vi "mono_radar.vi"(7 "Sensor Connections":T1(array[cluster])) -> (0 "error out":errorcluster, 1 "radar_data_cube":csg[][][](array[numeric]), 2 "Sensor Connections Out":T1(array[cluster]), 3 "connection ID out":refnum<k5>)   [LabVIEW 2018]
panel:
  in  "n_sweeps":i32=64
  in  "n_elements":i32=8
  in  "samples_per_sweep":i32=825
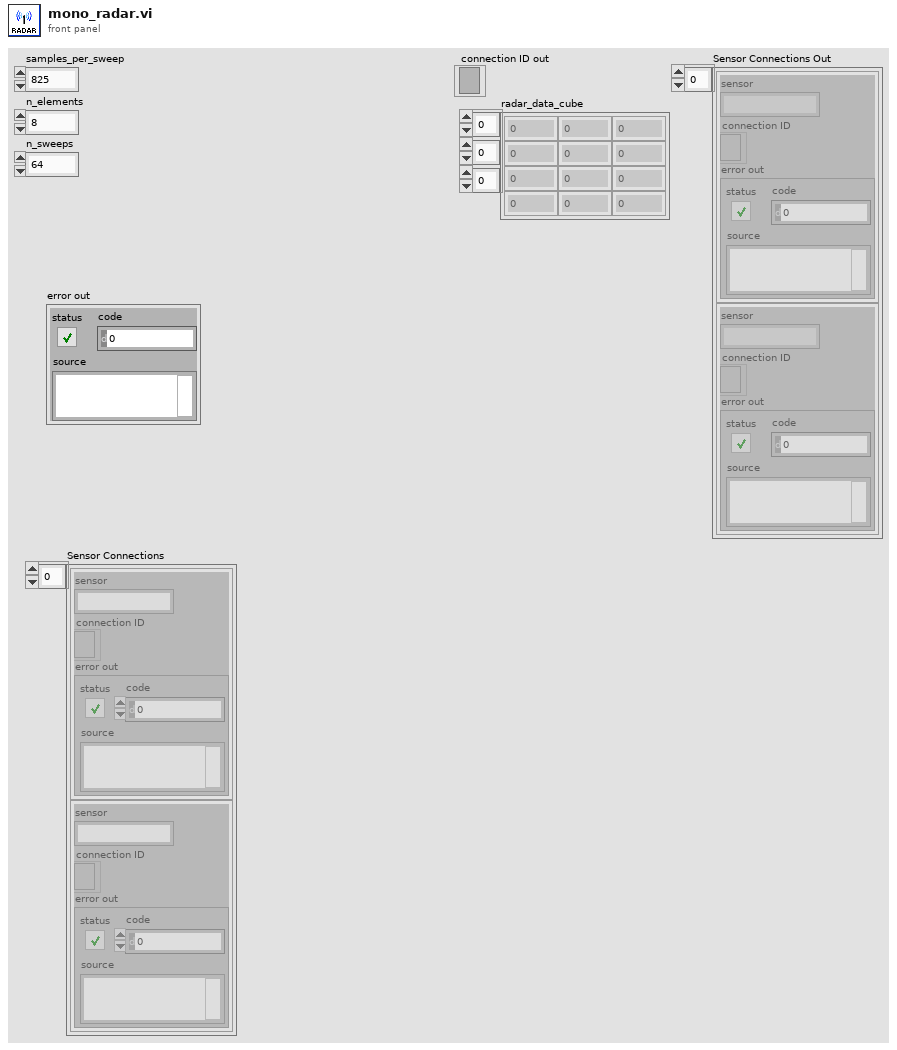
[diagram p1: front panel]
types:
  T1 = cluster{"sensor":string, "connection ID":refnum<k5>, "error out":errorcluster}[]
  T2 = cluster{"sensor":string, "connection ID":refnum<k5>, "error out":errorcluster}
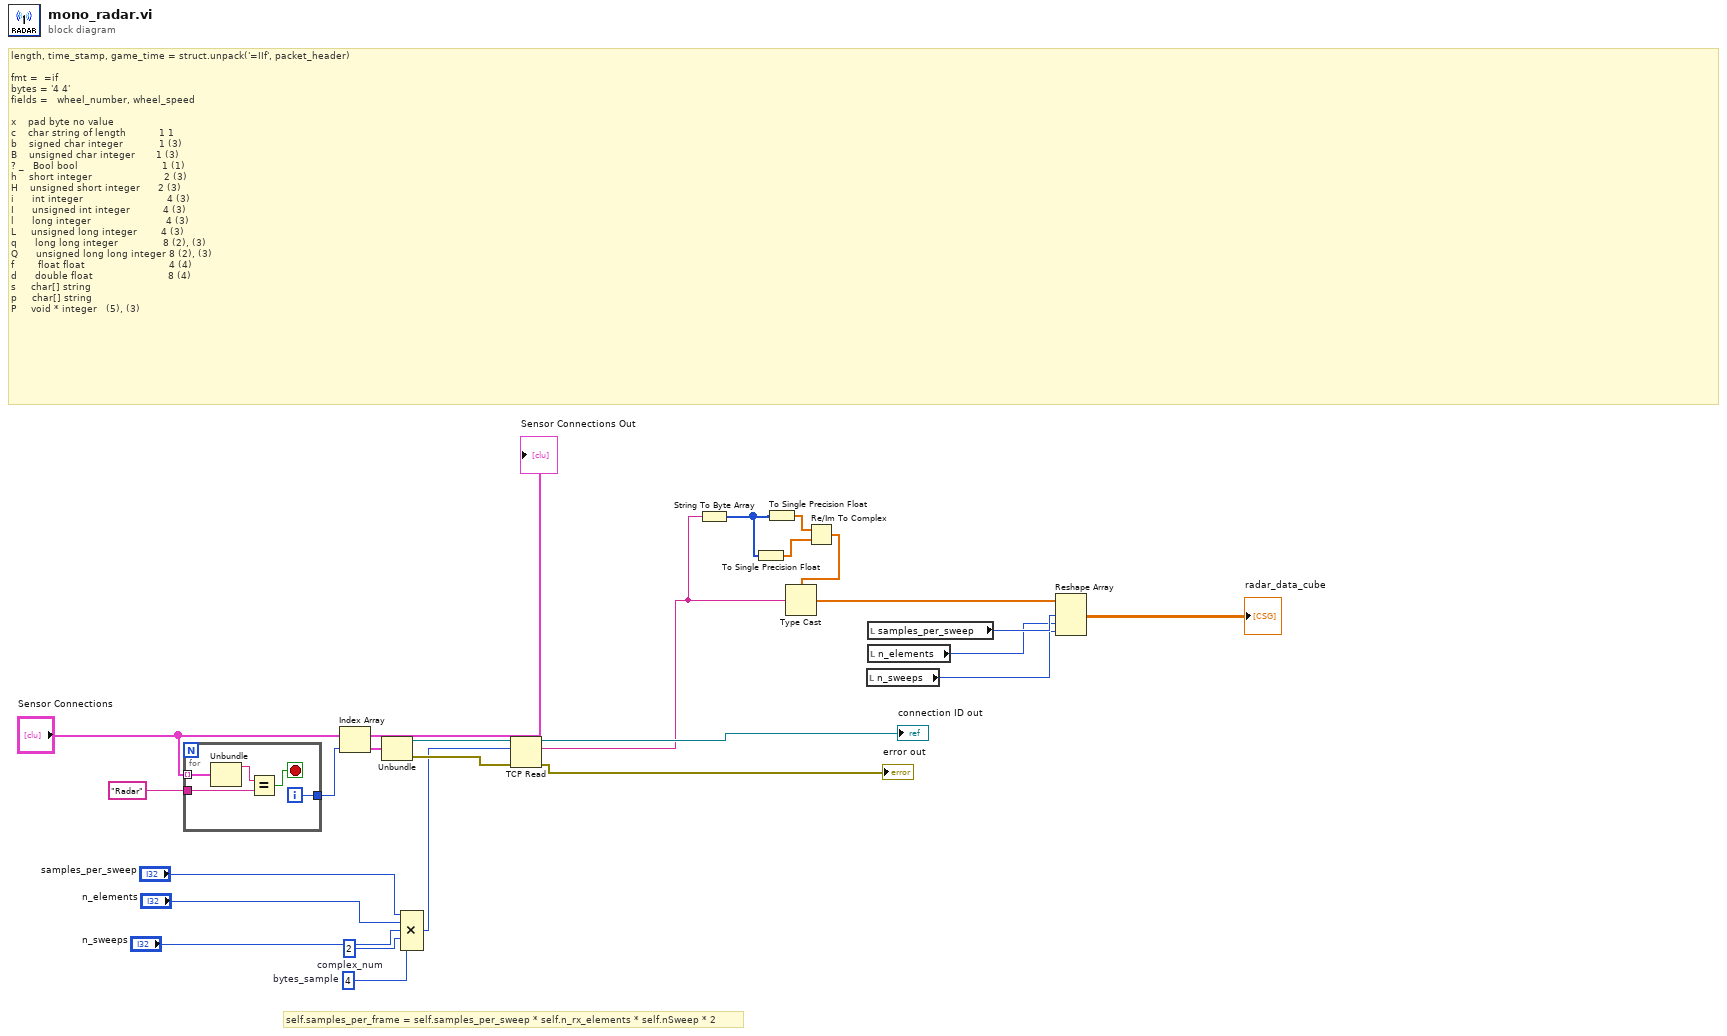
[diagram p0: block diagram]
diagram:
  w13 = 4  # bytes_sample
  w15 = 2  # complex_num
  # "self.samples_per_frame = self.samples_per_sweep * self.n_rx_elements * self.nSweep * 2"
  # "length, time_stamp, game_time = struct.unpack('=IIf', packet_header)\n\nfmt =  =if\nbytes = '4 4'\nfields =   wheel_number, wheel_speed\n\nx\t   pad byte\tno value\t \t \nc\t   char\tstring of length           1\t1\t \nb\t   signed char\tinteger\t           1\t(3)\nB\t   unsigned char\tinteger\t      1\t(3)\n?\t_   Bool\tbool\t                           1\t(1)\nh\t   short\tinteger\t                       2\t(3)\nH\t   unsigned short\tinteger\t     2\t(3)\ni\t     int\tinteger\t                           4\t(3)\nI\t     unsigned int\tinteger\t          4\t(3)\nl     \tlong\tinteger\t                        4\t(3)\nL\t    unsigned long\tinteger\t       4\t(3)\nq     \tlong long\tinteger\t              8\t(2), (3)\nQ\t     unsigned long long\tinteger\t8\t(2), (3)\nf       \tfloat\tfloat\t                           4\t(4)\nd     \tdouble\tfloat\t                        8\t(4)\ns\t    char[]\tstring\t \t \np\t    char[]\tstring\t \t \nP\t    void *\tinteger\t \t(5), (3)"
  n1 = for {
    tunnel: "Sensor Connections" -> [w29] mode=indexing
    tunnel: "Radar" -> [w27]
    tunnel: [w25] -> w22
    i -> [w25]
    stop <- w26 stop-if-true
    n2 = Unbundle(w29) -> ("sensor"=w28:string)  [unwired: 2 out]
    n3 = Equal?(x=w28, y=w27) -> (x = y?=w26:bool)
  }
  n4 = Index Array(array="Sensor Connections", index=w22) -> (element=w24:T2)
  n5 = Unbundle(w24) -> ("connection ID"=w20:refnum<k5>, "error out"=w19:errorcluster)  [unwired: 1 out]
  n6 = Compound Arithmetic op=MULTIPLY("samples_per_sweep", "n_elements", "n_sweeps", w15, w13) -> (w14:i32)
  n7 = TCP Read(connection ID=w20, bytes to read=w14, error in (no error)=w19) -> (connection ID out=→"connection ID out":refnum<k5>, data out=w10:string, error out=→"error out":errorcluster)  [unwired: 2 in]
  n8 = String To Byte Array(string=w10) -> (unsigned byte array=w9:u8[])
  n9 = To Single Precision Float(number=w9) -> (single precision float=w7:sgl[])
  n10 = To Single Precision Float(number=w9) -> (single precision float=w8:sgl[])
  n11 = Re/Im To Complex(1:w7, 2:w8) -> (0:w6:csg[])
  n12 = Type Cast(type=w6, x=w10) -> (*(type *) &x=w5:csg[])
  n13 = local read "n_sweeps"() -> (w2:i32)
  n14 = local read "samples_per_sweep"() -> (w4:i32)
  n15 = local read "n_elements"() -> (w3:i32)
  n16 = Reshape Array(w5, w4, w3, w2) -> (→"radar_data_cube":csg[][][])
  "Sensor Connections Out" <- "Sensor Connections"
